vi "gCode.vi"(8 "F":dbl, 9 "?":cluster{"X":dbl, "Y":dbl, "Z":dbl}, 11 "gCode":T1) -> (3 "String":string)   [LabVIEW 2017]
uses:
  controls/gCodeControl.ctl
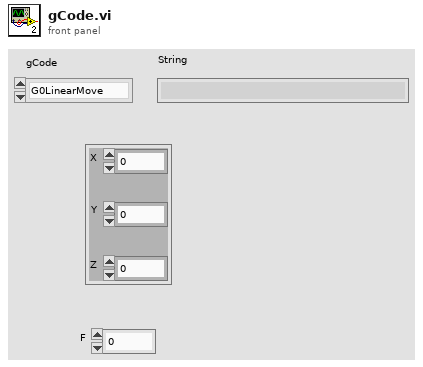
[diagram p1: front panel]
types:
  T1 = typedef "gCodeControl.ctl" = enum16{"G0LinearMove", "G1XY", "G1LinearMove", "G2Arc", "G4Dwell", "G20InchUnit", "G21MilliUnit", "G28AutoHome", "G92SetPosition", "G91RelativePos"}
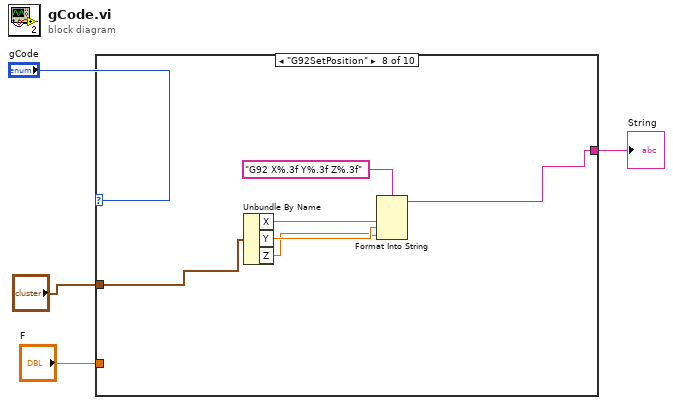
[diagram p0: block diagram]
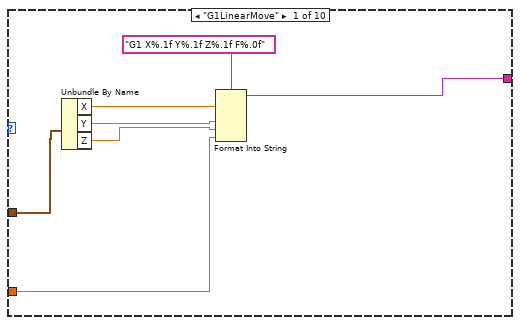
[diagram p2: hidden frame]
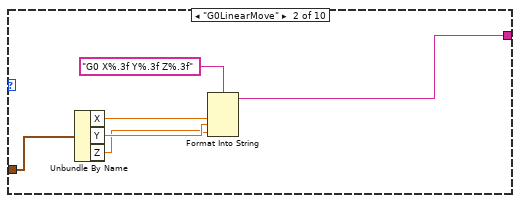
[diagram p3: hidden frame]
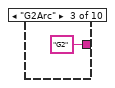
[diagram p4: hidden frame]
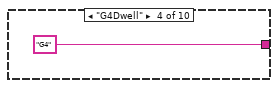
[diagram p5: hidden frame]
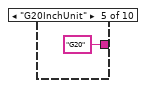
[diagram p6: hidden frame]
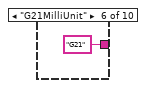
[diagram p7: hidden frame]
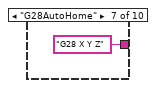
[diagram p8: hidden frame]
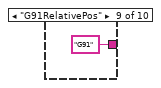
[diagram p9: hidden frame]
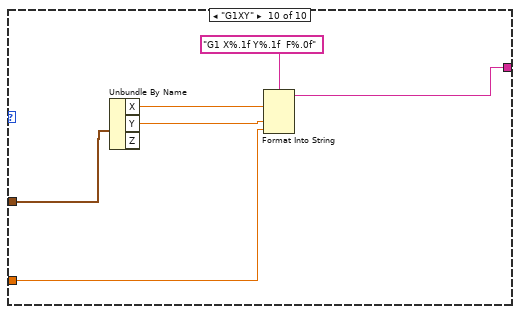
[diagram p10: hidden frame]
diagram:
  n1 = case shown="\"G92SetPosition\"" "gCode" {
    tunnel: [w7 w13 "G2" ("String") "G4" ("String") "G20" ("String") "G21" ("String") "G28 X Y Z" ("String") w24 "G91" ("String") w32] -> w3
    tunnel: "?" -> [w6 w16 _ _ _ _ _ w25 _ w31]
    tunnel: "F" -> [w5 _ _ _ _ _ _ _ _ w30]
    frame "G1LinearMove" {
      n2 = Unbundle By Name(w6) -> ("X"=w10:dbl, "Y"=w9:dbl, "Z"=w8:dbl)
      n3 = Format Into String(format string="G1 X%.1f Y%.1f Z%.1f F%.0f", w10, w9, w8, w5) -> (resulting string=w7:string)  [unwired: 2 in, 1 out]
    }
    frame "G0LinearMove" {
      n4 = Unbundle By Name(w16) -> ("X"=w15:dbl, "Y"=w14:dbl, "Z"=w12:dbl)
      n5 = Format Into String(format string="G0 X%.3f Y%.3f Z%.3f", w15, w14, w12) -> (resulting string=w13:string)  [unwired: 2 in, 1 out]
    }
    frame "G2Arc" {
    }
    frame "G4Dwell" {
    }
    frame "G20InchUnit" {
    }
    frame "G21MilliUnit" {
    }
    frame "G28AutoHome" {
    }
    frame "G92SetPosition" {
      n6 = Unbundle By Name(w25) -> ("X"=w27:dbl, "Y"=w26:dbl, "Z"=w23:dbl)
      n7 = Format Into String(format string="G92 X%.3f Y%.3f Z%.3f", w27, w26, w23) -> (resulting string=w24:string)  [unwired: 2 in, 1 out]
    }
    frame "G91RelativePos" {
    }
    frame "G1XY" {
      n8 = Unbundle By Name(w31) -> ("X"=w34:dbl, "Y"=w33:dbl)  [unwired: 1 out]
      n9 = Format Into String(format string="G1 X%.1f Y%.1f  F%.0f", w34, w33, w30) -> (resulting string=w32:string)  [unwired: 2 in, 1 out]
    }
  }
  "String" <- w3
